vi "Quaternion_Equals.vi"(9 "Other Quaternion":T1={"R"=1.0, "V"=[0.0, 0.0, 0.0]}, 11 "Quaternion":T1={"R"=1.0, "V"=[0.0, 0.0, 0.0]}) -> (3 "Equal":bool)   [LabVIEW 2019, in "Trajectory_Library.lvlib"]
doc: "Checks equality between this Quaternion and another object.\n\nParameters:\n - Quaternion - The quaternion data cluster.\n - Other Quaternion - The other quaternion data cluster.\n\nReturns:\n - Equal - Returns TRUE if both quaternions are equal."
uses:
  Trajectory_Library.lvlib
  TypeDef/QUATERNION.ctl
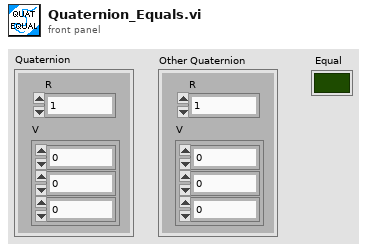
[diagram p1: front panel]
types:
  T1 = typedef "Trajectory_Library.lvlib/QUATERNION.ctl" = cluster{"R":dbl, "V":dbl[]}
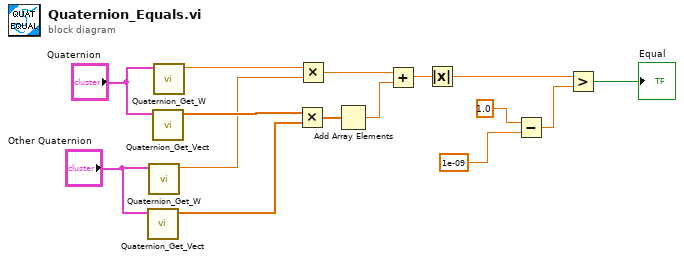
[diagram p0: block diagram]
diagram:
  n1 = call "Quaternion_Get_Vect.vi"("Quaternion"="Other Quaternion") -> ("Vector"=w1:dbl[])  [unwired: 10 in]
  n2 = call "Quaternion_Get_W.vi"("Quaternion"="Other Quaternion") -> ("W"=w2:dbl)  [unwired: 10 in]
  n3 = call "Quaternion_Get_Vect.vi"("Quaternion"="Quaternion") -> ("Vector"=w3:dbl[])  [unwired: 10 in]
  n4 = call "Quaternion_Get_W.vi"("Quaternion"="Quaternion") -> ("W"=w4:dbl)  [unwired: 10 in]
  n5 = Multiply(x=w3, y=w1) -> (x*y=w15:dbl[])
  n6 = Multiply(x=w4, y=w2) -> (x*y=w14:dbl)
  n7 = Add Array Elements(numeric array=w15) -> (sum=w13:dbl)
  n8 = Add(x=w14, y=w13) -> (x+y=w12:dbl)
  n9 = Absolute Value(x=w12) -> (abs(x)=w11:dbl)
  n10 = Subtract(x=1.0, y=1e-09) -> (x-y=w8:dbl)
  n11 = Greater?(x=w11, y=w8) -> (0:→"Equal":bool)
